vi "Get Version.vi"(8 "error in (no error)":errorcluster, 11 "VISA resource name":refnum<visa-resource-name>) -> (0 "error out":errorcluster, 2 "Version":i32(ring) items=["R1.03", "R2.01", "R2.02", "R2.03", "R3.01"], 3 "VISA resource name out":refnum<visa-resource-name>)   [LabVIEW 2020, in "Yokogawa GX Series.lvlib"]
uses:
  <instrlib>/Yokogawa GX Series/Yokogawa GX Series.lvlib
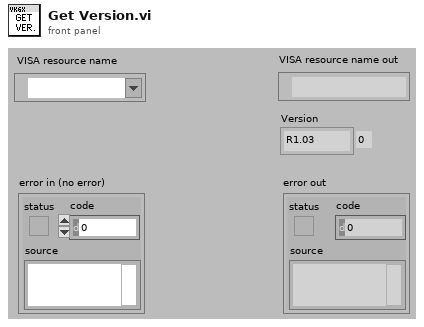
[diagram p1: front panel]
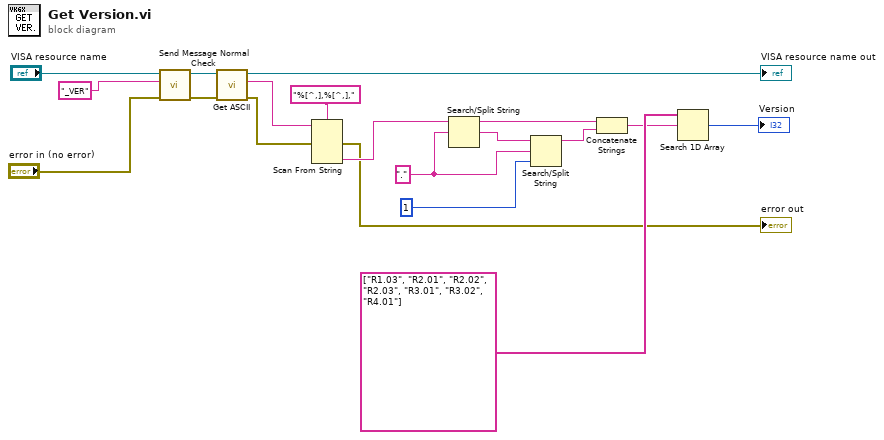
[diagram p0: block diagram]
diagram:
  w10 = "."
  n1 = call <instrlib>:"Send Message Normal Check.vi"("error in (no error)"="error in (no error)", "Send Message (\"\")"="_VER" ("書き込みバッファ"), "VISA resource name"="VISA resource name") -> ("error out"=w15:errorcluster, "VISA resource name out"=w16:refnum<visa-resource-name>)  [unwired: 3 in, 4 out]
  n2 = call <instrlib>:"Get ASCII.vi"("error in (no error)"=w15, "VISA resource name"=w16) -> ("error out"=w12:errorcluster, "ASCII Data"=w14:string, "VISA resource name out"=→"VISA resource name out":refnum<visa-resource-name>)  [unwired: 7 in]
  n3 = Scan From String(format string="%[^,],%[^,],", input string=w14, error in=w12) -> (error out=→"error out":errorcluster, output 2=w11:string)  [unwired: 1 in, 5 out]
  n4 = Search/Split String(string=w11, search string/char (-)=w10) -> (substring before match=w8:string, match + rest of string=w2:string)  [unwired: 1 in, 1 out]
  n5 = Search/Split String(string=w2, search string/char (-)=w10, offset (0)=1) -> (substring before match=w7:string)  [unwired: 2 out]
  n6 = Concatenate Strings(w8, w7) -> (w3:string)
  n7 = Search 1D Array(1D array=string[] ["R1.03", "R2.01", "R2.02", "R2.03", "R3.01", "R3.02", "R4.01"], element=w3) -> (index of element=→"Version":i32)  [unwired: 1 in]
